vi "Read Address Recursive Access.vi"(8 "error in (no error)":errorcluster, 11 "Simple Tree Queue Mailman in":refnum<class "Simple Tree Queue Mailman.lvclass">) -> (0 "error out":errorcluster, 2 "Address":i32[](array[numeric]), 3 "Simple Tree Queue Mailman out":refnum<class "Simple Tree Queue Mailman.lvclass">)   [LabVIEW 2024, in "Simple Tree Queue Mailman.lvclass"]
uses:
  Simple Tree Queue Mailman.lvclass
  Simple Tree Queue Mailman.lvclass/Simple Tree Queue Mailman.ctl
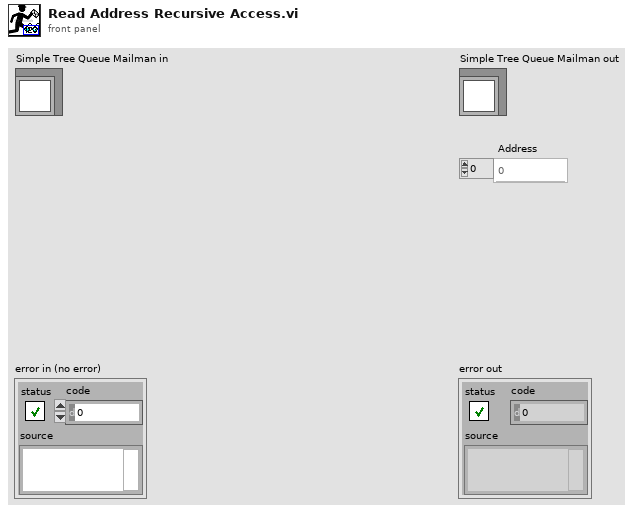
[diagram p1: front panel]
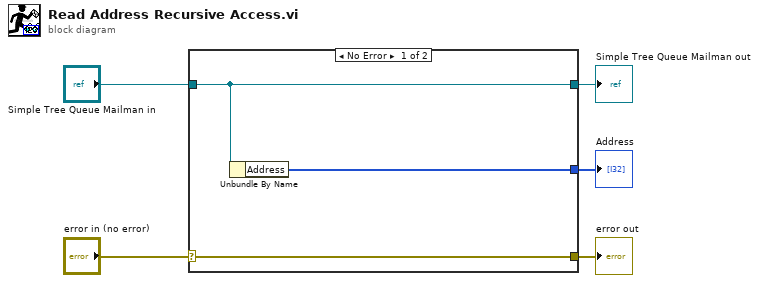
[diagram p0: block diagram]
diagram:
  n1 = case shown="No Error" "error in (no error)" {
    selector: "error in (no error)" -> [w8 w9]
    tunnel: [w8 w9] -> w4
    tunnel: [w7 w10] -> w2
    tunnel: "Simple Tree Queue Mailman in" -> [w7 w10]
    tunnel: [w6 _] -> w1
    frame No Error {
      n2 = Unbundle By Name(w7) -> ("Address"=w6:i32[])
    }
    frame Error {
    }
  }
  "error out" <- w4
  "Simple Tree Queue Mailman out" <- w2
  "Address" <- w1
